vi "gui.vi"() -> ()   [LabVIEW 2016]
uses:
  <vilib>/Instr/_visa.llb/VISA Configure Serial Port (Instr).vi
panel:
  out "Waveform Chart":i16(graph)
  out "Angle feedback (°)":i16(knob) scale=-180.0..180.0
  in  "Angle Set (°)":i16
  in  "Stop":bool
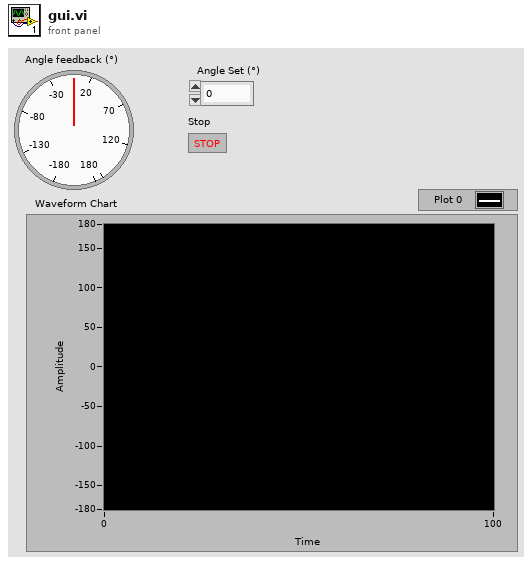
[diagram p1: front panel]
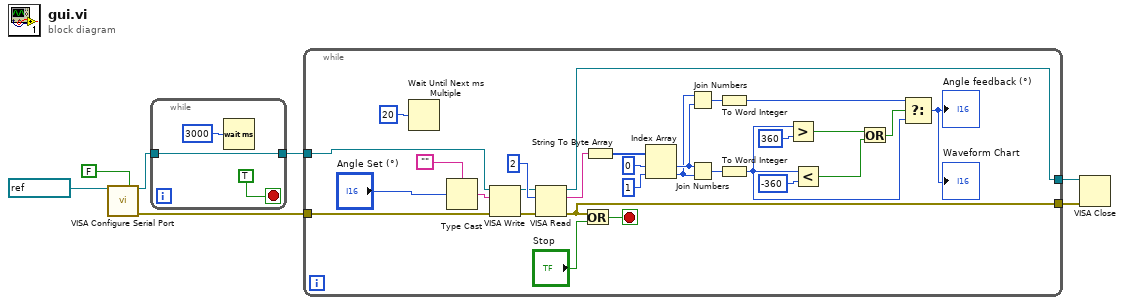
[diagram p0: block diagram]
diagram:
  n1 = call-poly "VISA Configure Serial Port"("VISA resource name"=refnum<visa-resource-name> "COM6", "Enable Termination\nChar (T)"=FALSE ("Enable Termination\nChar (T)")) -> ("VISA resource name out"=w5:refnum<visa-resource-name>, "error out"=w3:errorcluster)  [unwired: 12 in]
  n2 = while {
    tunnel: [w10] -> w4
    tunnel: w5 -> [w10]
    stop <- TRUE stop-if-true
    n3 = Wait (ms)(milliseconds to wait=u32 3000) -> ()  [unwired: 1 out]
  }
  n4 = while {
    tunnel: w4 -> [w39]
    tunnel: w3 -> [w37]
    tunnel: [w26] -> w2
    tunnel: [w23] -> w1
    stop <- w35 stop-if-true
    n5 = Wait Until Next ms Multiple(millisecond multiple=u32 20 ("milliseconds to wait")) -> ()  [unwired: 1 out]
    n6 = Type Cast(type="", x="Angle Set (°)") -> (*(type *) &x=w38:string)
    n7 = VISA Write(VISA resource name=w39, write buffer=w38, error in (no error)=w37) -> (VISA resource name out=w24:refnum<visa-resource-name>, error out=w27:errorcluster)  [unwired: 1 out]
    n8 = VISA Read(VISA resource name=w24, byte count=u32 2, error in (no error)=w27) -> (VISA resource name out=w23:refnum<visa-resource-name>, read buffer=w31:string, error out=w26:errorcluster)  [unwired: 1 out]
    n9 = Or(x=w26, y="Stop") -> (x .or. y?=w35:bool)
    n10 = String To Byte Array(string=w31) -> (unsigned byte array=w30:u8[])
    n11 = Index Array(array=w30, index #1=0 ("index"), index #2=1 ("index")) -> (element #1=w18:u8, element #2=w17:u8)
    n12 = Join Numbers(hi=w17, lo=w18) -> ((hi.lo)=w16:u16)
    n13 = Join Numbers(hi=w18, lo=w17) -> ((hi.lo)=w25:u16)
    n14 = To Word Integer(number=w16) -> (16bit integer=w15:i16)
    n15 = To Word Integer(number=w25) -> (16bit integer=w14:i16)
    n16 = Greater?(x=w14, y=i16 360) -> (0:w19:bool)
    n17 = Less?(x=w14, y=i16 -360) -> (x < y?=w20:bool)
    n18 = Or(x=w19, y=w20) -> (x .or. y?=w13:bool)
    n19 = Select(t=w15, s=w13, f=w14) -> (s? t:f=→"Angle feedback (°)" →"Waveform Chart":i16)
  }
  n20 = VISA Close(VISA resource name=w1, error in (no error)=w2) -> ()  [unwired: 1 out]
